vi "Create Message.vi"   [LabVIEW 2015, in "Car Wash.lvlib" / "AMC.lvlib"]
doc: "Creates an AMC message, which can be passed to Send Message.vi."
uses:
  AMC.lvlib
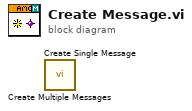
[diagram p0: block diagram]
diagram:
  n1 = call "Create Multiple Messages.vi"() -> ()  [unwired: 14 in, 2 out]
  n2 = call "Create Single Message.vi"() -> ()  [unwired: 14 in, 2 out]
